vi "Add Through Points.vi"(4 "Side":T1=enum."right", 7 "ByPass":bool=TRUE, 8 "error in":errorcluster, 10 "Goal":dbl[](array[numeric])) -> (0 "error out":errorcluster, 2 "Goal":dbl[](array[numeric]))   [LabVIEW 2013]
uses:
  ROS/Code/SubVIs/BaxterSide.ctl
  Arm Globals.vi
  ROS/Code/Console/Servers/ServerSubs/(nist) Arm Globals.vi
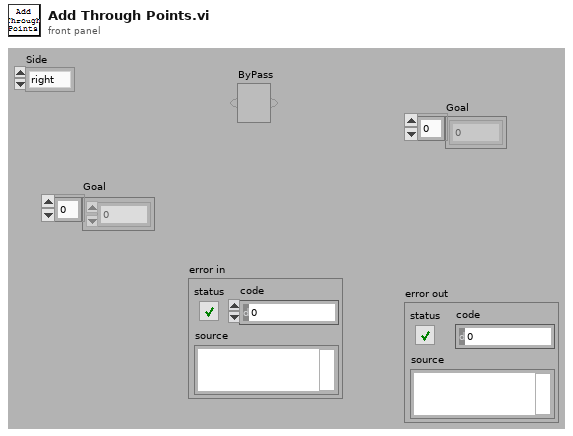
[diagram p1: front panel]
types:
  T1 = typedef "BaxterSide.ctl" = enum16{"left", "right"}
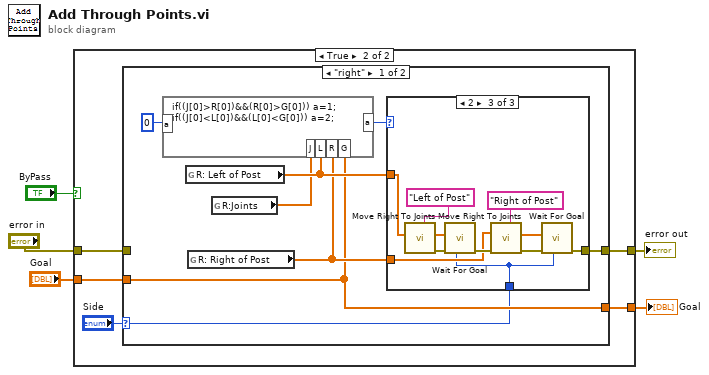
[diagram p0: block diagram]
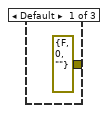
[diagram p3: hidden frame]
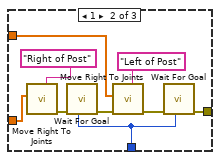
[diagram p4: hidden frame]
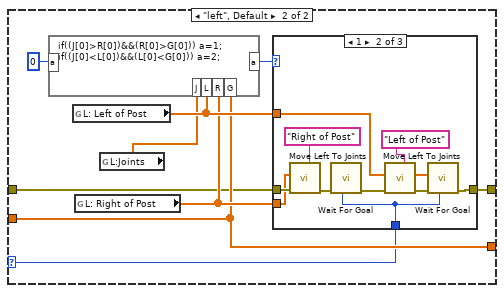
[diagram p5: hidden frame]
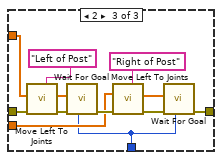
[diagram p7: hidden frame]
diagram:
  n1 = case shown="True" "ByPass" {
    tunnel: "Goal" -> [w7 w12]
    tunnel: [w7 w10] -> w4
    tunnel: [w6 w8] -> w2
    tunnel: "error in" -> [w6 w9]
    frame False {
    }
    frame True {
      n2 = case shown="\"right\"" "Side" {
        selector: "Side" -> [w15 w45]
        tunnel: [w16 w46] -> w10
        tunnel: w12 -> [w16 w46]
        tunnel: w9 -> [_ w44]
        tunnel: [w14 w43] -> w8
        frame "right" {
          n3 = global read "Arm Globals.vi" "R: Left of Post"() -> (w18:dbl[])
          n4 = global read "Arm Globals.vi" "R: Right of Post"() -> (w17:dbl[])
          n5 = global read "(nist) Arm Globals.vi" "R:Joints"() -> (w13:dbl[])
          n6 = formula code="if((J[0]>R[0])&&(R[0]>G[0])) a=1;\nif((J[0]<L[0])&&(L[0]<G[0])) a=2;"("L"=w18, "R"=w17, "G"=w16, "J"=w13, "a"=0) -> ("a"=w19:i32)
          n7 = case shown="2" w19 {
            tunnel: w18 -> [_ w26 w36]
            tunnel: w17 -> [_ w30 w35]
            tunnel: w15 -> [_ w22 w33]
            tunnel: [errorcluster {"status"=FALSE, "code"=0, "source"=""} ("error out") w23 w34] -> w14
            frame Default {
            }
            frame 1 {
              n8 = call "Move Right To Joints.vi"("Label"="Right of Post", "Goal"=w30) -> ("error out"=w28:errorcluster)  [unwired: 8 in, 1 out]
              n9 = call "Wait For Goal.vi"("Side"=w22, "error in"=w28) -> ("error out"=w27:errorcluster)  [unwired: 8 in, 1 out]
              n10 = call "Move Right To Joints.vi"("Label"="Left of Post", "error in"=w27, "Goal"=w26) -> ("error out"=w25:errorcluster)  [unwired: 7 in, 1 out]
              n11 = call "Wait For Goal.vi"("Side"=w22, "error in"=w25) -> ("error out"=w23:errorcluster)  [unwired: 8 in, 1 out]
            }
            frame 2 {
              n12 = call "Move Right To Joints.vi"("Label"="Left of Post", "Goal"=w36) -> ("error out"=w40:errorcluster, "Goal"=w32:dbl[])  [unwired: 8 in]
              n13 = call "Wait For Goal.vi"("Side"=w33, "error in"=w40, "Goal"=w32) -> ("error out"=w39:errorcluster)  [unwired: 7 in, 1 out]
              n14 = call "Move Right To Joints.vi"("Label"="Right of Post", "error in"=w39, "Goal"=w35) -> ("error out"=w38:errorcluster, "Goal"=w31:dbl[])  [unwired: 7 in]
              n15 = call "Wait For Goal.vi"("Side"=w33, "error in"=w38, "Goal"=w31) -> ("error out"=w34:errorcluster)  [unwired: 7 in, 1 out]
            }
          }
        }
        frame "left", Default {
          n16 = global read "Arm Globals.vi" "L: Left of Post"() -> (w48:dbl[])
          n17 = global read "Arm Globals.vi" "L: Right of Post"() -> (w47:dbl[])
          n18 = global read "(nist) Arm Globals.vi" "L:Joints"() -> (w42:dbl[])
          n19 = formula code="if((J[0]>R[0])&&(R[0]>G[0])) a=1;\nif((J[0]<L[0])&&(L[0]<G[0])) a=2;"("L"=w48, "R"=w47, "G"=w46, "J"=w42, "a"=0) -> ("a"=w49:i32)
          n20 = case shown="1" w49 {
            tunnel: w48 -> [_ w55 w69]
            tunnel: w47 -> [_ w54 w68]
            tunnel: w45 -> [_ w61 w66]
            tunnel: [w51 w62 w67] -> w43
            tunnel: w44 -> [w51 w60 w65]
            frame Default {
            }
            frame 1 {
              n21 = call "Move Left To Joints.vi"("Label"="Right of Post", "error in"=w60, "Goal"=w54) -> ("error out"=w59:errorcluster)  [unwired: 7 in, 1 out]
              n22 = call "Wait For Goal.vi"("Side"=w61, "error in"=w59) -> ("error out"=w58:errorcluster)  [unwired: 8 in, 1 out]
              n23 = call "Move Left To Joints.vi"("Label"="Left of Post", "error in"=w58, "Goal"=w55) -> ("error out"=w57:errorcluster, "Goal"=w56:dbl[])  [unwired: 7 in]
              n24 = call "Wait For Goal.vi"("Side"=w61, "error in"=w57, "Goal"=w56) -> ("error out"=w62:errorcluster)  [unwired: 7 in, 1 out]
            }
            frame 2 {
              n25 = call "Move Left To Joints.vi"("Label"="Left of Post", "error in"=w65, "Goal"=w69) -> ("error out"=w73:errorcluster, "Goal"=w64:dbl[])  [unwired: 7 in]
              n26 = call "Wait For Goal.vi"("Side"=w66, "error in"=w73, "Goal"=w64) -> ("error out"=w72:errorcluster)  [unwired: 7 in, 1 out]
              n27 = call "Move Left To Joints.vi"("Label"="Right of Post", "error in"=w72, "Goal"=w68) -> ("error out"=w71:errorcluster, "Goal"=w63:dbl[])  [unwired: 7 in]
              n28 = call "Wait For Goal.vi"("Side"=w66, "error in"=w71, "Goal"=w63) -> ("error out"=w67:errorcluster)  [unwired: 7 in, 1 out]
            }
          }
        }
      }
    }
  }
  "Goal" <- w4
  "error out" <- w2
